vi "(18) part 2 que.vi"() -> ()   [LabVIEW 2025]
panel:
  in  "Numeric 4":dbl
  in  "Numeric 3":dbl
  out "Numeric 2":dbl
  in  "Numeric":dbl
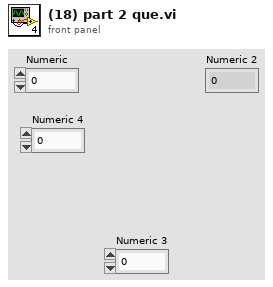
[diagram p1: front panel]
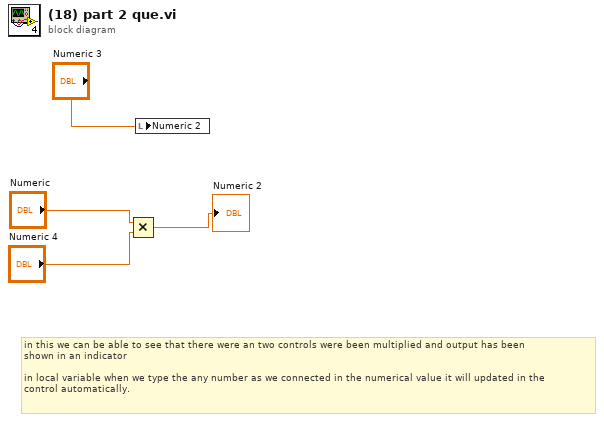
[diagram p0: block diagram]
diagram:
  # "in this we can be able to see that there were an two controls were been multiplied and output has been \nshown in an indicator \n\nin local variable when we type the any number as we connected in the numerical value it will updated in the \ncontrol automatically."
  n1 = Multiply(x="Numeric", y="Numeric 4") -> (x*y=→"Numeric 2":dbl)
  n2 = local write "Numeric 2"("Numeric 3") -> ()
